vi "Insight_Sweep_Direction.vi"(8 "error in (no error)":errorcluster, 9 "Mode (Read / Write)":enum8{"Write", "Read"}(ring), 10 "WL Sweep Direction":T1(ring)=enum."Bidirectional_Increase", 11 "telnet connection":T2) -> (0 "error out":errorcluster, 1 "WL Sweep Direction?":T1(ring), 2 "response data":string, 3 "telnet connection out":T2)   [LabVIEW 2011]
doc: "Insight Photonic Solutions\n\nThis VI sets or queries the direction of change of wavelength during a sweep of the laser. Options are Increasing (wavelength), Decreasing (wavelength), Bidirectional_Increase (sweep increasing, then decreasing wavelength), and Bidirectional_Decrease (sweep decreasing, then increasing wavelength).\n\nver 1.0 - original release"
uses:
  Telnet Session.ctl
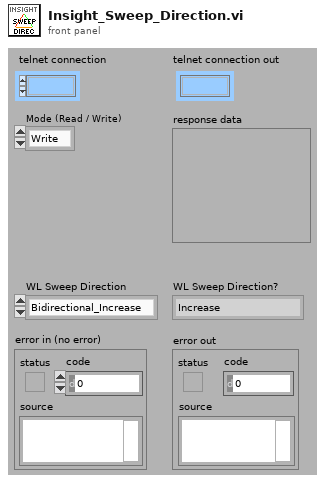
[diagram p1: front panel]
types:
  T1 = enum16{"Increase", "Decrease", "Bidirectional_Increase", "Bidirectional_Decrease"}
  T2 = typedef "Telnet Session.ctl" = refnum<k1>
  T3 = enum16{"INCReasing", "DECReasing", "BINCreasing", "BDECreasing"}
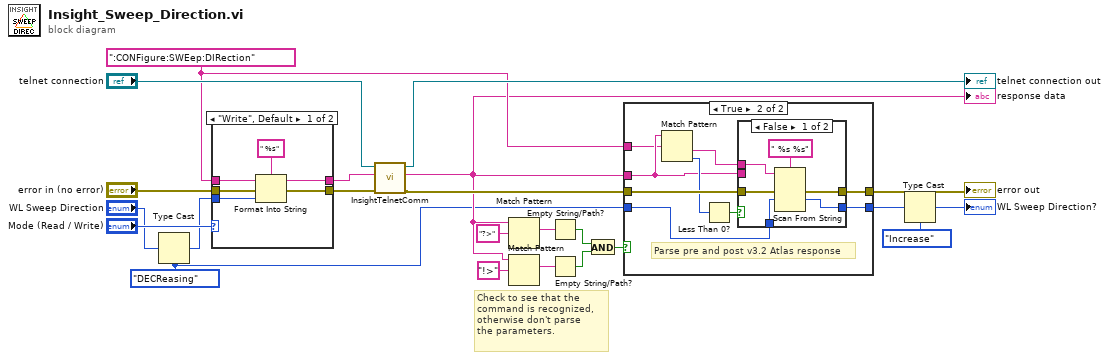
[diagram p0: block diagram]
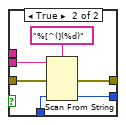
[diagram p3: hidden frame]
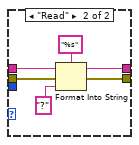
[diagram p4: hidden frame]
diagram:
  w4 = T3."DECReasing" ("Trigger Edge")
  w8 = ":CONFigure:SWEep:DIRection" ("String")
  # "Check to see that the \ncommand is recognized,\notherwise don't parse \nthe parameters."
  n1 = Type Cast(type=w4, x="WL Sweep Direction") -> (*(type *) &x=w5:T3)
  n2 = case shown="\"Write\", Default" "Mode (Read / Write)" {
    tunnel: [w29 w31] -> w21
    tunnel: "error in (no error)" -> [w28 w30]
    tunnel: w8 -> [w27 w33]
    tunnel: w5 -> [w24 _]
    tunnel: [w25 w32] -> w20
    frame "Write", Default {
      n3 = Format Into String(format string=" %s", initial string=w27, error in=w28, w24) -> (resulting string=w25:string, error out=w29:errorcluster)
    }
    frame "Read" {
      n4 = Format Into String(format string="%s", initial string=w33, error in=w30, "?" ("input 1")) -> (resulting string=w32:string, error out=w31:errorcluster)
    }
  }
  n5 = call "InsightTelnetComm.vi"("error in"=w21, "write buffer (\"\")"=w20, "telnet connection"="telnet connection") -> ("error out"=w10:errorcluster, "response data"=w7:string, "telnet  connection out"=→"telnet connection out":T2)  [unwired: 4 in]
  "response data" <- w7
  n6 = Match Pattern(string=w7, regular expression="?>") -> (match substring=w13:string)  [unwired: 1 in, 3 out]
  n7 = Match Pattern(string=w7, regular expression="!>") -> (match substring=w14:string)  [unwired: 1 in, 3 out]
  n8 = Empty String/Path?(string/path=w13) -> (empty?=w16:bool)
  n9 = Empty String/Path?(string/path=w14) -> (empty?=w17:bool)
  n10 = And(x=w16, y=w17) -> (x .and. y?=w11:bool)
  n11 = case shown="True" w11 {
    tunnel: [w37 w44] -> w9
    tunnel: w10 -> [w37 w43]
    tunnel: w7 -> [_ w40]
    tunnel: [w36 w45] -> w3
    tunnel: w8 -> [_ w39]
    tunnel: w4 -> [w36 w38]
    frame False {
    }
    frame True {
      # "Parse pre and post v3.2 Atlas response"
      n12 = Match Pattern(string=w40, regular expression=w39) -> (after substring=w41:string, offset past match=w42:i32)  [unwired: 1 in, 2 out]
      n13 = Less Than 0?(x=w42) -> (x < 0?=w46:bool)
      n14 = case shown="False" w46 {
        tunnel: w41 -> [w51 _]
        tunnel: w40 -> [_ w57]
        tunnel: [w52 w58] -> w44
        tunnel: [w49 w56] -> w45
        tunnel: w43 -> [w48 w55]
        tunnel: w38 -> [w47 w54]
        frame False {
          n15 = Scan From String(format string=" %s %s" ("f"), input string=w51, error in=w48, default 1=w47) -> (error out=w52:errorcluster, output 1=w49:T3)  [unwired: 3 in, 2 out]
        }
        frame True {
          n16 = Scan From String(format string="%[^(](%d)", input string=w57, error in=w55, default 2=w54) -> (error out=w58:errorcluster, output 2=w56:T3)  [unwired: 3 in, 2 out]
        }
      }
    }
  }
  "error out" <- w9
  n17 = Type Cast(type=T1."Increase" ("WL Sweep Direction"), x=w3) -> (*(type *) &x=→"WL Sweep Direction?":T1)
